vi "ELOG_TimestampFormat_Get.vi"(8 "error in (no error)":errorcluster, 11 "OXY_SCPI Reseource In":refnum<visa-resource-name>) -> (0 "error out":errorcluster, 1 "communication_data":T2, 2 "Timestamp Format":T1, 3 "OXY_SCPI Reseource Out":refnum<visa-resource-name>)   [LabVIEW 2018, in "OXYGEN.lvlib"]
doc: "Queries the currently configured timestamp format."
uses:
  OXYGEN.lvlib
  TypeDefs/Cluster_RawCommData.ctl
  TypeDefs/Enum_ELOGtimeFormats.ctl
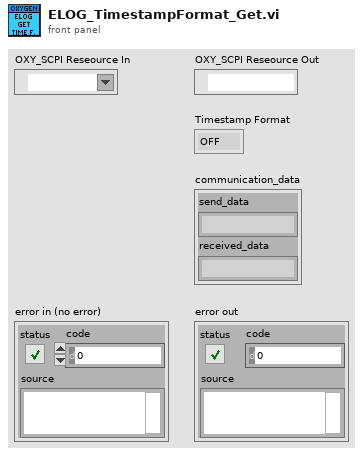
[diagram p1: front panel]
types:
  T1 = typedef "OXYGEN.lvlib/Enum_ELOGtimeFormats.ctl" = enum16{"OFF", "REL", "ELOG", "ABS"}
  T2 = typedef "OXYGEN.lvlib/Cluster_RawCommData.ctl" = cluster{"send_data":string, "received_data":string}
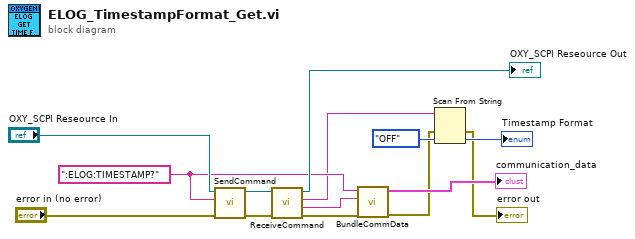
[diagram p0: block diagram]
diagram:
  w6 = ":ELOG:TIMESTAMP?" ("string")
  n1 = call "SendCommand.vi"("error in (no error)"="error in (no error)", "String to Send"=w6, "OXY_SCPI Reseource In"="OXY_SCPI Reseource In") -> ("error out"=w10:errorcluster, "OXY_SCPI Reseource Out"=w11:refnum<visa-resource-name>)  [unwired: 7 in]
  n2 = call "ReceiveCommand.vi"("error in (no error)"=w10, "OXY_SCPI Reseource In"=w11) -> ("error out"=w8:errorcluster, "received Data with Header"=w7:string, "received Data"=w5:string, "OXY_SCPI Reseource Out"=→"OXY_SCPI Reseource Out":refnum<visa-resource-name>)  [unwired: 6 in]
  n3 = call "BundleCommData.vi"("error in (no error)"=w8, "received_data"=w7, "send_data"=w6) -> ("error out"=w1:errorcluster, "communication_data"=→"communication_data":T2)  [unwired: 7 in]
  n4 = Scan From String "Scan From String"(input string=w5, error in=w1, default 1=Enum_ELOGtimeFormats."OFF" ("Timestamp Format")) -> (error out=→"error out":errorcluster, output 1=→"Timestamp Format":T1)  [unwired: 2 in, 2 out]
